vi "Analogue Read.vi"(8 "error in":errorcluster, 11 "task/channels in":refnum<k21>) -> (0 "error out":errorcluster, 1 "RPM":i32[](array[knob]) scale=0.0..200.0, 2 "measured force":dbl[](array[numeric]), 3 "task out":refnum<k21>)   [LabVIEW 2021]
uses:
  <vilib>/Analysis/3filter.llb/Filter Passband Type.ctl
  <vilib>/DAQmx/read.llb/DAQmx Read (Analog 1D DBL NChan 1Samp).vi
  <vilib>/DAQmx/miscellaneous.llb/DAQmx Fill In Error Info.vi
  <vilib>/ptbypt/NI_PtbyPt.lvlib
  <vilib>/Analysis/NI_AALBase.lvlib
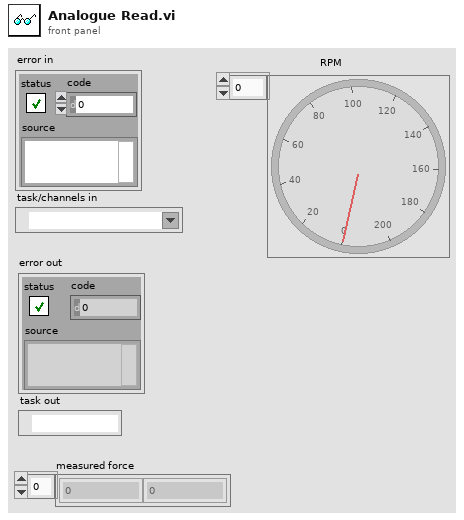
[diagram p1: front panel]
types:
  T1 = typedef "NI_AALBase.lvlib/Filter Passband Type.ctl" = enum32{"Lowpass", "Highpass", "Bandpass", "Bandstop"}
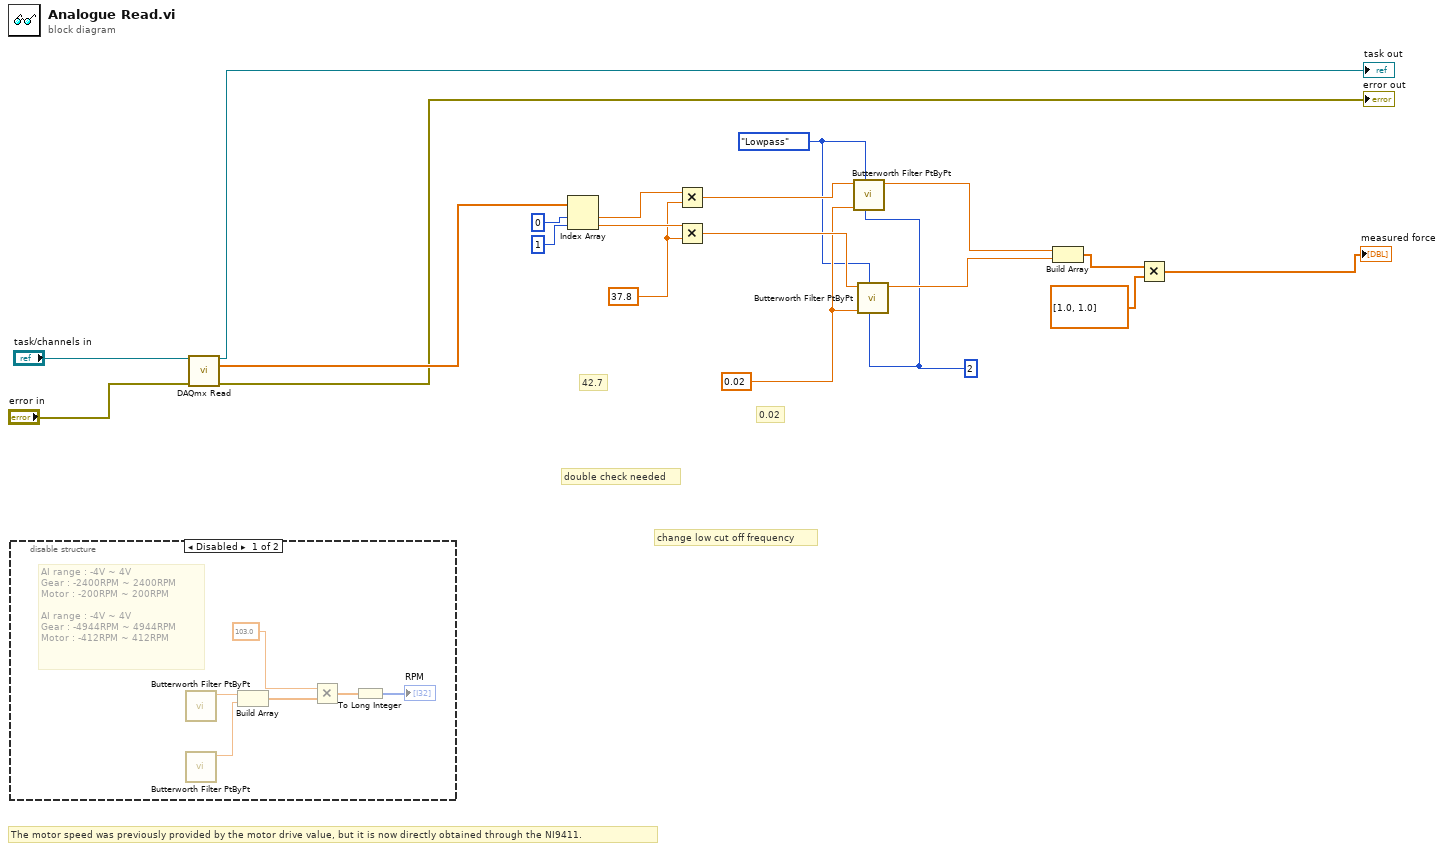
[diagram p0: block diagram]
diagram:
  w5 = 2 ("order")
  w7 = 0.02 ("low cutoff freq: fl")
  w4 = 37.8 ("y")
  w6 = Filter_Passband_Type."Lowpass" ("filter type")
  # "0.02"
  # "42.7"
  # "The motor speed was previously provided by the motor drive value, but it is now directly obtained through the NI9411."
  # "change low cut off frequency"
  # "double check needed"
  n1 = disable-structure shown="Disabled" {
    frame Disabled {
      # "AI range : -4V ~ 4V\nGear : -2400RPM ~ 2400RPM\nMotor : -200RPM ~ 200RPM\n\nAI range : -4V ~ 4V\nGear : -4944RPM ~ 4944RPM\nMotor : -412RPM ~ 412RPM"
      n2 = call <vilib>:"Butterworth Filter PtByPt.vi"() -> ("Filtered x"=w24:dbl)  [unwired: 9 in, 1 out]
      n3 = call <vilib>:"Butterworth Filter PtByPt.vi"() -> ("Filtered x"=w25:dbl)  [unwired: 9 in, 1 out]
      n4 = Build Array(w24, w25) -> (w26:dbl[])
      n5 = Multiply(x=103.0, y=w26) -> (x*y=w23:dbl[])
      n6 = To Long Integer(number=w23) -> (32bit integer=→"RPM":i32[])
    }
    frame Enabled {
    }
  }
  n7 = call-poly <vilib>:"DAQmx Read.vi"("task/channels in"="task/channels in", "error in"="error in") -> ("task out"=→"task out":refnum<k21>, "data"=w9:dbl[], "error out"=→"error out":errorcluster)  [unwired: 11 in]
  n8 = Index Array(array=w9, index #1=0 ("index"), index #2=1 ("index")) -> (element #1=w12:dbl, element #2=w11:dbl)
  n9 = Multiply(x=w12, y=w4) -> (x*y=w13:dbl)
  n10 = Multiply(x=w11, y=w4) -> (x*y=w10:dbl)
  n11 = call <vilib>:"Butterworth Filter PtByPt.vi"("order"=w5, "filter type"=w6, "low cutoff freq: fl"=w7, "x"=w13) -> ("Filtered x"=w18:dbl)  [unwired: 5 in, 1 out]
  n12 = call <vilib>:"Butterworth Filter PtByPt.vi"("order"=w5, "filter type"=w6, "low cutoff freq: fl"=w7, "x"=w10) -> ("Filtered x"=w17:dbl)  [unwired: 5 in, 1 out]
  n13 = Build Array(w18, w17) -> (w3:dbl[])
  n14 = Multiply(x=w3, y=dbl[] [1.0, 1.0]) -> (x*y=→"measured force":dbl[])
